vi "Dig.vi"(8 "Error In":errorcluster, 10 "Selection List[]":refnum<vi>[](array[refnum]), 11 "VI In":refnum<vi>) -> (0 "Error Out":errorcluster, 2 "Change Made?":bool, 3 "VI Out":refnum<vi>)   [LabVIEW 2017, in "Eulogy.lvlib"]
doc: "A VI script that encloses a selection of code in a Diagram Disable Contional structure, creates a duplicate of the original code to be refactored for the Enabled frame, adds an \"Original\" and \"Refactored\" subdiagram label to each frame, respectively, and adds a bookmark with \"RIP\", the DoD (Date of Death), and grave digger (programmer) as the structure's label.\n\nBy default, today's date is used as the DoD and the application's user name is used for the grave digger."
uses:
  Eulogy.lvlib
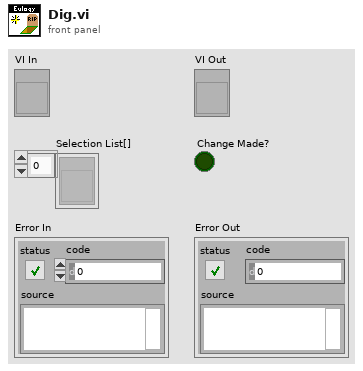
[diagram p1: front panel]
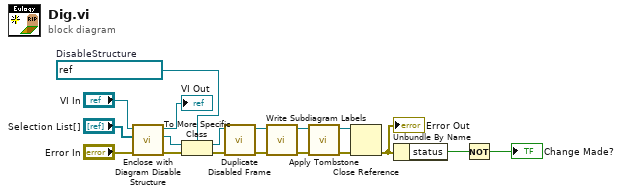
[diagram p0: block diagram]
diagram:
  w17 = refnum<vi> refnum  # DisableStructure
  n1 = call "Enclose with Diagram Disable Structure.vi"("Error In"="Error In", "Selection List[]"="Selection List[]", "VI In"="VI In") -> ("Error Out"=w11:errorcluster, "Diagram Disable Structure"=w18:refnum<vi>, "VI Out"=→"VI Out":refnum<vi>)  [unwired: 6 in]
  n2 = To More Specific Class(target class=w17, reference=w18, error in=w11) -> (specific class reference=w16:refnum<vi>, error out=w15:errorcluster)
  n3 = call "Duplicate Disabled Frame.vi"("Error In"=w15, "DisableStructure In"=w16) -> ("Error Out"=w14:errorcluster, "DisableStructure Out"=w13:refnum<vi>)  [unwired: 8 in]
  n4 = call "Write Subdiagram Labels.vi"("Error In"=w14, "DisableStructure In"=w13) -> ("Error Out"=w6:errorcluster, "DisableStructure Out"=w12:refnum<vi>)  [unwired: 8 in]
  n5 = call "Apply Tombstone.vi"("Error In"=w6, "Grave In"=w12) -> ("Error Out"=w10:errorcluster, "Grave Out"=w9:refnum<vi>)  [unwired: 8 in]
  n6 = Close Reference(reference=w9, error in (no error)=w10) -> (error out=w3:errorcluster)
  "Error Out" <- w3
  n7 = Unbundle By Name(w3) -> ("status"=w2:bool)
  n8 = Not(x=w2) -> (.not. x?=→"Change Made?":bool)
